vi "AIT 1553 Bus Page.vi"(8 "error in (no error)":errorcluster, 11 "Node Ptr":T1 format="%.0x") -> (0 "error out":errorcluster)   [LabVIEW 2013]
uses:
  <vilib>/NI Veristand/Custom Device API/Custom Device Item Ref.ctl
  Controls and Global/Global.vi
  <vilib>/NI Veristand/Custom Device API/Get Item Property (Path).vi
  <vilib>/NI Veristand/Custom Device API/Get Item Property (U16).vi
  <vilib>/NI Veristand/Custom Device API/Get Item Property (String).vi
  <vilib>/NI Veristand/Custom Device API/Custom Device API.lvlib
  AIT 664 Custom Device.lvlib
  <vilib>/NI Veristand/Custom Device API/Set Item Property (String).vi
panel:
  out "Bus Number":u16
  in  "RefreshDB":bool
  in  "Warning text":string="WARNING: The database has changed since import. If you attempt to run this system definition an error may occur. Consider refreshing the database import."
  out "Warn Icon":bool
  out "Database File":path
  in  "Header":cluster{"Section Name":string}={"Section Name"="AIT 1553 Bus"}
  in  "Description":string
  in  "Name":string
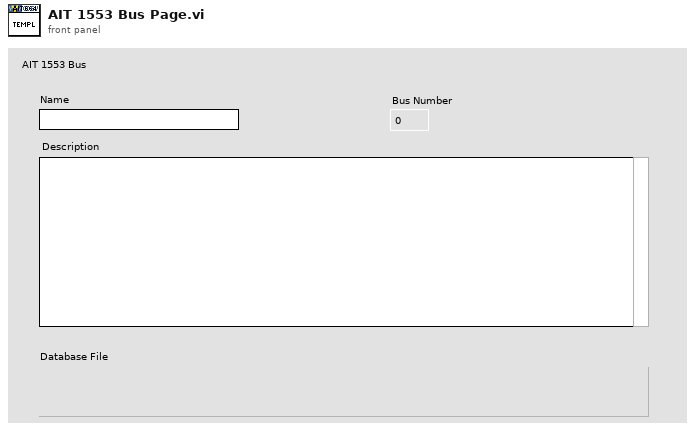
[diagram p1: front panel]
types:
  T1 = typedef "Custom Device API.lvlib/Custom Device Item Ref.ctl" = u64
  T2 = typedef "Custom Device API.lvlib/Custom Device Item Info.ctl" = cluster{"Name":string, "Is Channel":bool, "GUID":string, "Is Waveform":bool}
  T3 = typedef "Custom Device API.lvlib/Custom Device Commands.ctl" = enum16{"Default", "Item renamed", "Shutdown", "Dynamic button pressed"}
  T4 = typedef "AIT 664 Custom Device.lvlib/Refresh Match Settings.ctl" = cluster{"Ch by name?":bool, "Lbl by name?":bool}
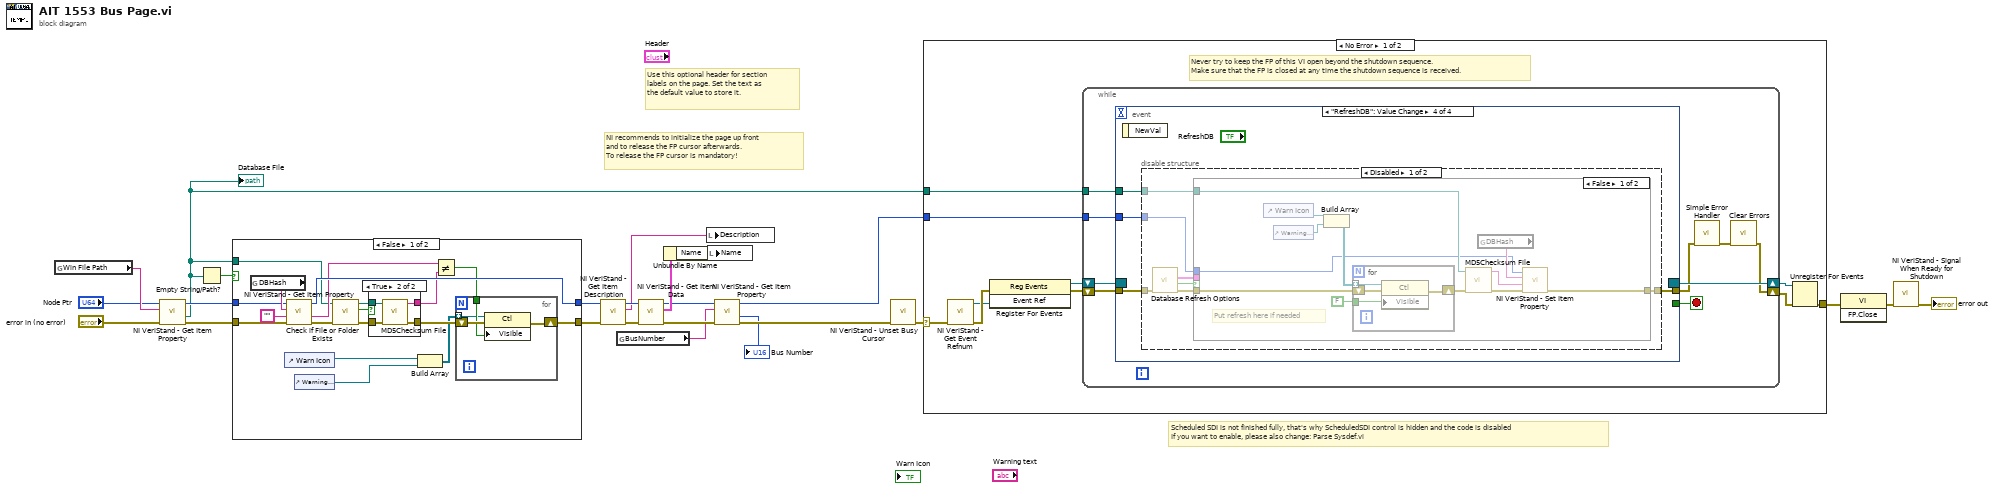
[diagram p0: block diagram]
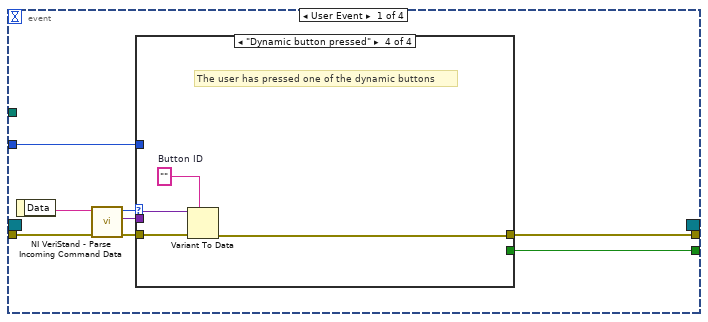
[diagram p4: hidden frame]
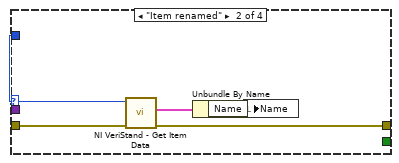
[diagram p6: hidden frame]
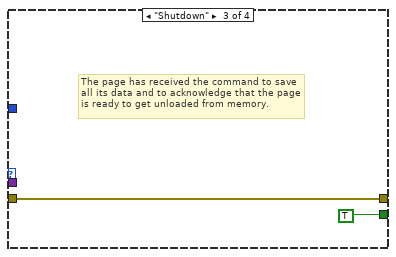
[diagram p7: hidden frame]
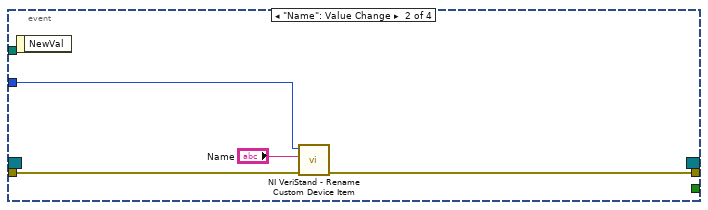
[diagram p8: hidden frame]
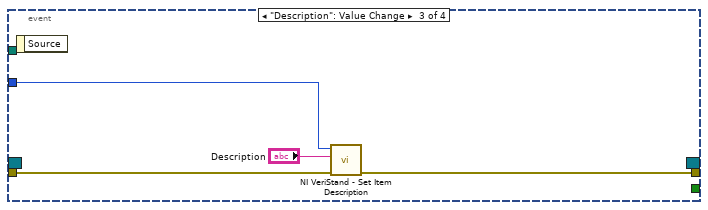
[diagram p9: hidden frame]
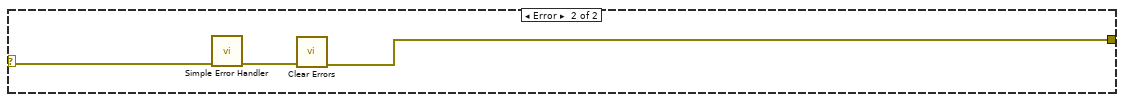
[diagram p12: hidden frame]
diagram:
  # "Scheduled SDI is not finished fully, that's why ScheduledSDI control is hidden and the code is disabled\nIf you want to enable, please also change: Parse Sysdef.vi"
  # "Use this optional header for section labels on the page. Set the text as the default value to store it."
  # "NI recommends to initialize the page up front\nand to release the FP cursor afterwards.\nTo release the FP cursor is mandatory!"
  n1 = global read "Global.vi" "Win File Path"() -> (w15:string)
  n2 = call-poly <vilib>:"NI VeriStand - Get Item Property.vi"("error in (no error)"="error in (no error)", "Property Name"=w15, "Item Ref in"="Node Ptr") -> ("error out"=w13:errorcluster, "Value"=w11:path, "Item Ref out"=w12:T1)  [unwired: 5 in, 1 out]
  "Database File" <- w11
  n3 = Empty String/Path?(string/path=w11) -> (empty?=w14:bool)
  n4 = case shown="False" w14 {
    tunnel: w13 -> [w39 w53]
    tunnel: [w30 w53] -> w7
    tunnel: [w38 w52] -> w8
    tunnel: w12 -> [w40 w52]
    tunnel: w11 -> [w26 _]
    frame False {
      n5 = global read "Global.vi" "DBHash"() -> (w41:string)
      n6 = control-ref of="Warn Icon"() -> (w32:refnum<vi>)
      n7 = call-poly <vilib>:"NI VeriStand - Get Item Property.vi"("error in (no error)"=w39, "Default Value"="", "Property Name"=w41, "Item Ref in"=w40) -> ("error out"=w27:errorcluster, "Value"=w36:string, "Item Ref out"=w38:T1)  [unwired: 4 in, 1 out]
      n8 = control-ref of="Warning text"() -> (w33:refnum<vi>)
      n9 = call <vilib>:"Check if File or Folder Exists.vi"("error in (no error)"=w27, "path"=w26) -> ("error out"=w29:errorcluster, "file or folder exists?"=w25:bool, "dup path"=w28:path)  [unwired: 7 in]
      n10 = case shown="True" w25 {
        tunnel: [_ w47] -> w37
        tunnel: [w43 w46] -> w35
        tunnel: w29 -> [w43 w45]
        tunnel: w28 -> [_ w44]
        frame False {
        }
        frame True {
          n11 = call <vilib>:"MD5Checksum File.vi"("error in (no error)"=w45, "Path"=w44) -> ("error out"=w46:errorcluster, "MD5 message-digest"=w47:string)  [unwired: 8 in]
        }
      }
      n12 = Build Array(w32, w33) -> (w31:refnum<vi>[])
      n13 = Not Equal?(x=w36, y=w37) -> (x != y?=w34:bool)
      n14 = for {
        shift-right: [w50] -> w30
        shift-left: w35 -> [w51]
        tunnel: w34 -> [w49]
        tunnel: w31 -> [w48] mode=indexing
        n15 = property class="Ctl"(reference=w48, error in=w51, "Visible"=w49) -> (error out=w50:errorcluster)  [unwired: 1 out]
      }
    }
    frame True {
    }
  }
  n16 = call <vilib>:"NI VeriStand - Get Item Description.vi"("error in (no error)"=w7, "Item Ref in"=w8) -> ("error out"=w18:errorcluster, "Description"=w19:string, "Item Ref out"=w20:T1)  [unwired: 7 out]
  n17 = global read "Global.vi" "BusNumber"() -> (w2:string)
  n18 = call <vilib>:"NI VeriStand - Get Item Data.vi"("error in (no error)"=w18, "Item Ref in"=w20) -> ("error out"=w5:errorcluster, "Item Info"=w17:T2, "Item Ref out"=w6:T1)  [unwired: 7 out]
  n19 = Unbundle By Name(w17) -> ("Name"=w16:string)
  n20 = local write "Description"(w19) -> ()
  n21 = local write "Name"(w16) -> ()
  n22 = call-poly <vilib>:"NI VeriStand - Get Item Property.vi"("error in (no error)"=w5, "Property Name"=w2, "Item Ref in"=w6) -> ("error out"=w3:errorcluster, "Value"=→"Bus Number":u16, "Item Ref out"=w4:T1)  [unwired: 5 in, 1 out]
  n23 = call <vilib>:"NI VeriStand - Unset Busy Cursor.vi"("error in (no error)"=w3) -> ("error out"=w21:errorcluster)  [unwired: 10 out]
  n24 = case shown="No Error" w21 {
    selector: w21 -> [w55 w132]
    tunnel: [w60 w130] -> w24
    tunnel: w4 -> [w56 _]
    tunnel: w11 -> [w54 _]
    frame No Error {
      # "Never try to keep the FP of this VI open beyond the shutdown sequence.\nMake sure that the FP is closed at any time the shutdown sequence is received."
      n25 = call <vilib>:"NI VeriStand - Get Event Refnum.vi"("error in (no error)"=w55) -> ("error out"=w63:errorcluster, "Event Ref"=w59:refnum<user-event>)  [unwired: 9 out]
      n26 = register-events(error in=w63, w59) -> (reference out=w57:refnum<event-registration>, error out=w58:errorcluster)  [unwired: 1 in]
      n27 = while {
        tunnel: w56 -> [w68]
        shift-right: [w65] -> w61
        shift-left: w58 -> [w71]
        shift-right: [w72] -> w62
        shift-left: w57 -> [w70]
        tunnel: w54 -> [w64]
        stop <- w69 stop-if-true
        n28 = event shown="[3] \"RefreshDB\": Value Change" {
          selector: w70 -> [_ _ _ _]
          dyn-events: [_ _ _ _] -> w72
          timeout: _ -> [_ _ _ _]
          tunnel: w71 -> [w80 w96 w99 w102]
          tunnel: [w76 _ _ _] -> w69
          tunnel: [w75 w95 w98 w101] -> w67
          tunnel: w68 -> [w74 w94 w100 w103]
          tunnel: w64 -> [_ _ _ w104]
          event User Event {
            n29 = event-data() -> ("Data"=w79:string)  [unwired: 1 out]
            n30 = call <vilib>:"NI VeriStand - Parse Incoming Command Data.vi"("error in (no error)"=w80, "Incoming data"=w79) -> ("error out"=w78:errorcluster, "Outgoing data"=w73:variant, "Action"=w77:T3)  [unwired: 7 out]
            n31 = case shown="\"Dynamic button pressed\"" w77 {
              tunnel: w78 -> [w81 w86 w87 w92]
              tunnel: [_ _ TRUE _] -> w76
              tunnel: [w81 w83 w87 w89] -> w75
              tunnel: w74 -> [_ w85 _ _]
              tunnel: w73 -> [_ _ _ w91]
              frame "Default", Default {
              }
              frame "Item renamed" {
                n32 = call <vilib>:"NI VeriStand - Get Item Data.vi"("error in (no error)"=w86, "Item Ref in"=w85) -> ("error out"=w83:errorcluster, "Item Info"=w84:T2)  [unwired: 8 out]
                n33 = Unbundle By Name(w84) -> ("Name"=w82:string)
                n34 = local write "Name"(w82) -> ()
              }
              frame "Shutdown" {
                # "The page has received the command to save all its data and to acknowledge that the page is ready to get unloaded from memory."
              }
              frame "Dynamic button pressed" {
                w90 = ""  # Button ID
                # "The user has pressed one of the dynamic buttons"
                n35 = Variant To Data(error in=w92, type=w90, Variant=w91) -> (error out=w89:errorcluster)  [unwired: 1 out]
              }
            }
          }
          event "Name": Value Change {
            n36 = event-data() -> ()  [unwired: 2 out]
            n37 = call <vilib>:"NI VeriStand - Rename Custom Device Item.vi"("error in (no error)"=w96, "New Name"="Name", "Item Ref in"=w94) -> ("error out"=w95:errorcluster)  [unwired: 1 in, 7 out]
          }
          event "Description": Value Change {
            n38 = event-data() -> ()  [unwired: 2 out]
            n39 = call <vilib>:"NI VeriStand - Set Item Description.vi"("error in (no error)"=w99, "Description"="Description", "Item Ref in"=w100) -> ("error out"=w98:errorcluster)  [unwired: 8 out]
          }
          event "RefreshDB": Value Change {
            n40 = event-data() -> ()  [unwired: 2 out]
            n41 = disable-structure shown="Disabled" {
              disable-tunnel: w104 -> [w111 _]
              disable-tunnel: w103 -> [w110 _]
              disable-tunnel: w102 -> [w106 w129]
              disable-tunnel: [w105 w129] -> w101
              frame Disabled {
                n42 = call "Database Refresh Options.vi"("error in (no error)"=w106) -> ("error out"=w109:errorcluster, "Cancelled?"=w108:bool, "Refresh Settings"=w107:T4)  [unwired: 8 in]
                n43 = case shown="False" w108 {
                  tunnel: [w114 w128] -> w105
                  tunnel: w109 -> [w112 w128]
                  tunnel: w111 -> [w115 _]
                  tunnel: w110 -> [w113 _]
                  tunnel: w107 -> [_ _]
                  frame False {
                    # "Put refresh here if needed"
                    n44 = control-ref of="Warn Icon"() -> (w119:refnum<vi>)
                    n45 = control-ref of="Warning text"() -> (w120:refnum<vi>)
                    n46 = Build Array(w119, w120) -> (w117:refnum<vi>[])
                    n47 = for {
                      shift-right: [w126] -> w118
                      shift-left: w112 -> [w127]
                      tunnel: w117 -> [w125] mode=indexing
                      tunnel: FALSE ("Visible") -> [w124]
                      n48 = property class="Ctl"(reference=w125, error in=w127, "Visible"=w124) -> (error out=w126:errorcluster)  [unwired: 1 out]
                    }
                    n49 = call <vilib>:"MD5Checksum File.vi"("error in (no error)"=w118, "Path"=w115) -> ("error out"=w123:errorcluster, "MD5 message-digest"=w122:string)  [unwired: 8 in]
                    n50 = global read "Global.vi" "DBHash"() -> (w121:string)
                    n51 = call-poly <vilib>:"NI VeriStand - Set Item Property.vi"("error in (no error)"=w123, "Value"=w122, "Property Name"=w121, "Item Ref in"=w113) -> ("error out"=w114:errorcluster)  [unwired: 5 in, 2 out]
                  }
                  frame True {
                  }
                }
              }
              frame Enabled {
              }
            }
          }
        }
        n52 = call <vilib>:"Simple Error Handler.vi"("error in (no error)"=w67) -> ("error out"=w66:errorcluster)  [unwired: 1 in, 7 out]
        n53 = call <vilib>:"Clear Errors.vi"("error in (no error)"=w66) -> ("error out"=w65:errorcluster)  [unwired: 6 out]
      }
      n54 = Unregister For Events(event registration refnum=w62, error in=w61) -> (error out=w60:errorcluster)
    }
    frame Error {
      n55 = call <vilib>:"Simple Error Handler.vi"("error in (no error)"=w132) -> ("error out"=w131:errorcluster)  [unwired: 1 in, 7 out]
      n56 = call <vilib>:"Clear Errors.vi"("error in (no error)"=w131) -> ("error out"=w130:errorcluster)  [unwired: 6 out]
    }
  }
  n57 = invoke class="VI" method="FP.Close"(error in=w24) -> (error out=w23:errorcluster)  [unwired: 2 in, 2 out]
  n58 = call <vilib>:"NI VeriStand - Signal When Ready for Shutdown.vi"("error in (no error)"=w23) -> ("error out"=→"error out":errorcluster)  [unwired: 10 out]
